vi "4Pi 4Pi Modes - Mode Scan Counter.vi"(0 "Center Value":dbl=7.0, 2 "Action":T1, 7 "Mode":i32, 9 "Number of Steps":u16, 11 "Step Size":u16) -> (4 "Scan Done?":bool, 8 "Mode Amount":dbl, 15 "Current Mode":i32)   [LabVIEW 2016]
uses:
  4Pi 4Pi Modes - Controls/4Pi 4Pi Modes - Standard Counter Action.ctl
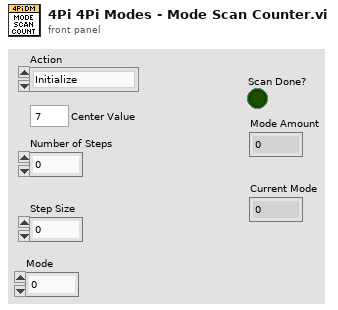
[diagram p1: front panel]
types:
  T1 = typedef "4Pi 4Pi Modes - Standard Counter Action.ctl" = enum16{"Initialize", "Update Count", "Get Count"}
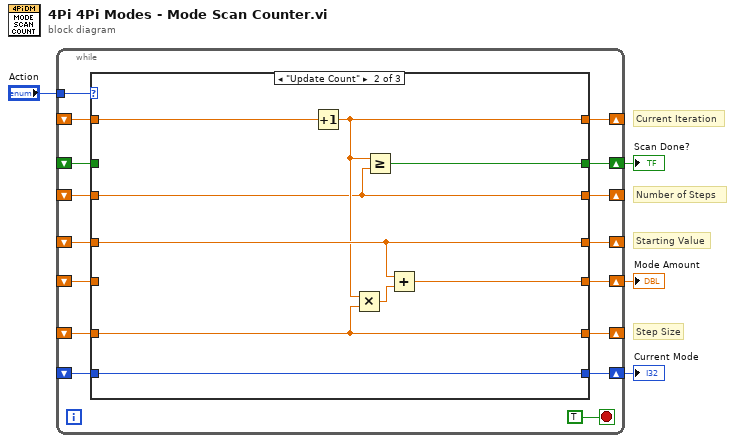
[diagram p0: block diagram]
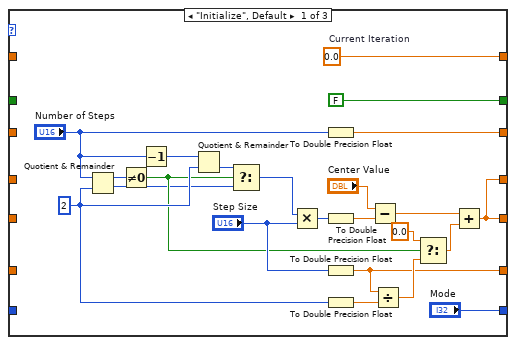
[diagram p2: hidden frame]
diagram:
  # "Starting Value"
  # "Current Iteration"
  # "Step Size"
  # "Number of Steps"
  n1 = while {
    tunnel: "Action" -> [w20]
    shift-right: [w19] -> _
    shift-left: _ -> [w15]
    shift-right: [w17] -> _
    shift-left: _ -> [w12]
    shift-right: [w18] -> _
    shift-left: _ -> [w14]
    shift-right: [w16] -> w2
    shift-left: _ -> [w13]
    shift-right: [w11] -> w3
    shift-left: _ -> [w10]
    shift-right: [w8] -> _
    shift-left: _ -> [w7]
    shift-right: [w6] -> w1
    shift-left: _ -> [w5]
    stop <- TRUE stop-if-true
    n2 = case shown="\"Update Count\"" w20 {
      tunnel: [w43 w46 w59] -> w19
      tunnel: [w26 w52 w56] -> w18
      tunnel: [w24 w45 w58] -> w17
      tunnel: [w22 w50 w57] -> w16
      tunnel: w15 -> [_ w47 w59]
      tunnel: w14 -> [_ w52 w56]
      tunnel: w13 -> [_ _ w57]
      tunnel: w12 -> [_ w45 w58]
      tunnel: [FALSE w49 w55] -> w11
      tunnel: w10 -> [_ _ w55]
      tunnel: [w22 w48 w54] -> w8
      tunnel: w7 -> [_ w48 w54]
      tunnel: ["Mode" w44 w53] -> w6
      tunnel: w5 -> [_ w44 w53]
      frame "Initialize", Default {
        w40 = u16 2 ("y")
        w43 = 0.0  # Current Iteration
        n3 = Quotient & Remainder(x="Number of Steps", y=w40) -> (x-y*floor(x/y)=w27:u16, floor(x/y)=w30:u16)
        n4 = Not Equal To 0?(x=w27) -> (x != 0?=w39:bool)
        n5 = Decrement(x="Number of Steps") -> (x-1=w28:u16)
        n6 = Quotient & Remainder(x=w28, y=w40) -> (floor(x/y)=w29:u16)  [unwired: 1 out]
        n7 = Select(t=w29, s=w39, f=w30) -> (s? t:f=w31:u16)
        n8 = Multiply(x=w31, y="Step Size") -> (x*y=w33:u16)
        n9 = To Double Precision Float(number="Number of Steps") -> (double precision float=w24:dbl)
        n10 = To Double Precision Float(number=w33) -> (double precision float=w34:dbl)
        n11 = To Double Precision Float(number="Step Size") -> (double precision float=w26:dbl)
        n12 = To Double Precision Float(number=w40) -> (double precision float=w41:dbl)
        n13 = Subtract(x="Center Value", y=w34) -> (x-y=w35:dbl)
        n14 = Divide(x=w26, y=w41) -> (x/y=w36:dbl)
        n15 = Select(t=0.0, s=w39, f=w36) -> (s? t:f=w37:dbl)
        n16 = Add(x=w35, y=w37) -> (x+y=w22:dbl)
      }
      frame "Update Count" {
        n17 = Increment(x=w47) -> (x+1=w46:dbl)
        n18 = Multiply(x=w46, y=w52) -> (x*y=w51:dbl)
        n19 = Greater Or Equal?(x=w46, y=w45) -> (x >= y?=w49:bool)
        n20 = Add(x=w48, y=w51) -> (x+y=w50:dbl)
      }
      frame "Get Count" {
      }
    }
  }
  "Scan Done?" <- w3
  "Mode Amount" <- w2
  "Current Mode" <- w1
